vi "Get Control Value and Type by Name.vi"(8 "错误输入（无错误）":errorcluster, 10 "Control Name":string, 11 "VI Ref":refnum<vi>) -> (0 "错误输出":errorcluster, 2 "Type Enum":T1, 3 "Control Value":variant)   [LabVIEW 2012, in "VIRef.lvlib"]
uses:
  VIRef.lvlib
  <vilib>/Utility/VariantDataType/Type.ctl
  <vilib>/Utility/VariantDataType/VariantType.lvlib
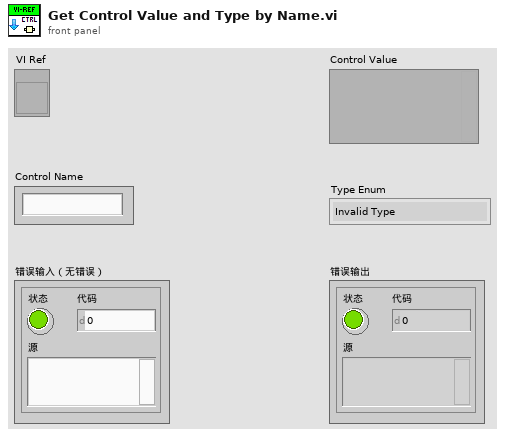
[diagram p1: front panel]
types:
  T1 = typedef "VariantType.lvlib/Type.ctl" = enum8{"Invalid Type", "Void", "I8", "I16", "I32", "I64", "U8", "U16", "U32", "U64", "Single Float", "Double Float", "Extended Float", "Single Complex", "Double Complex", "Extended Complex", "Enum U8", "Enum U16", "Enum U32", "Enum U64", "Single Float With Unit", "Double Float With Unit", "Extended Float With Unit", "Single Complex with Unit", "Double Complex with Unit", "Extended Complex with Unit", "Boolean", "String", "Path", "Picture", "Tag", "Array", "Cluster", "Variant", "LV Variant", "Waveform", "Timestamp", "Digital Waveform", "Digital Data", "ExpressData", "Refnum", "External Data", "VI", "Poly VI", "LabVIEW Class Instance", "Fixed Point"}
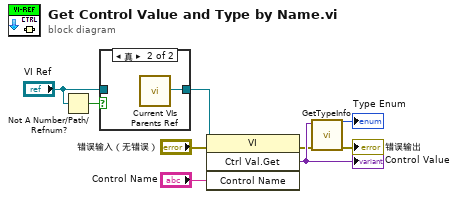
[diagram p0: block diagram]
diagram:
  n1 = Not A Number/Path/Refnum?(number/path/refnum="VI Ref") -> (NaN/Path/Refnum?=w9:bool)
  n2 = case shown="真" w9 {
    tunnel: [w10 w11] -> w7
    tunnel: "VI Ref" -> [w10 _]
    frame False {
    }
    frame True {
      n3 = call "Current VIs Parents Ref.vi"() -> ("Calling VI's Reference"=w11:refnum<vi>)  [unwired: 2 in]
    }
  }
  n4 = invoke class="VI" method="Ctrl Val.Get"(reference=w7, error in="错误输入（无错误）", "Control Name"="Control Name") -> (error out=w2:errorcluster, "Get Control Value Variant"=w4:variant)  [unwired: 1 in, 2 out]
  "Control Value" <- w4
  n5 = call <vilib>:"GetTypeInfo.vi"("error in (no error)"=w2, "Variant"=w4) -> ("error out"=→"错误输出":errorcluster, "Type Enum"=→"Type Enum":T1)  [unwired: 5 in, 3 out]
